vi "Top_Row.vi"(4 "NumRows":u32, 5 "Step In":i32) -> (1 "Step Out":i32)   [LabVIEW 2020]
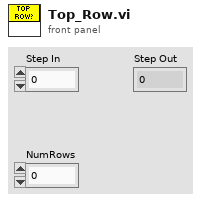
[diagram p1: front panel]
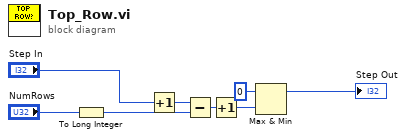
[diagram p0: block diagram]
diagram:
  n1 = To Long Integer(number="NumRows") -> (32bit integer=w5:i32)
  n2 = Increment(x="Step In") -> (x+1=w2:i32)
  n3 = Subtract(x=w2, y=w5) -> (x-y=w1:i32)
  n4 = Increment(x=w1) -> (x+1=w3:i32)
  n5 = Max & Min(x=0, y=w3) -> (max(x,y)=→"Step Out":i32)  [unwired: 1 out]
